vi "AlliGator Fit Method Benchmark.vi"() -> ()   [LabVIEW 2021, in "AlliGator Fit Method Benchmark.lvlib"]
doc: "Fit Method Benchmark GUI."
uses:
  AlliGator Fit Method Benchmark.lvlib
  AlliGator Fit Simulation Parameters.ctl
  AlliGator Decay Simulation Parameters.ctl
  Arrays/Array Statistics.ctl
  Fits/IRF(X)PSED/Decay Fit Options v4.ctl
  Fits/Decay Convolution/Decay Model.ctl
  Fits/Residual Type.ctl
  Fits/IRF(X)PSED/Fit Weights Type v2.ctl
  Fits/Non-linear Fitting Method v2.ctl
  Fits/Fit Calculation Method.ctl
  Fits/Non-linear Fitting Algorithm.ctl
  Decay Analysis/Decay Fit/AlliGator Decay Fit Parameter Constraints 2.ctl
  Fits/IRF(X)PSED/Decay Fit Parameters In List.ctl
  Fits/IRF(X)PSED/MLE Baseline Offset Type.ctl
  AlliGator Simulation Parameters.ctl
  AlliGator Simulation Parameters x Factors.ctl
  AlliGator FMB Histogram Options.ctl
  Graphs/XY Graph/XY Graph Refnum.ctl
  AlliGator FMB Q Element.ctl
  AlliGator FMB Q Event List.ctl
  AlliGator Simulation & Fit Options & Parameters.ctl
  Decay Fit Parameter Map/AlliGator Decay Fit Options & Parameters v4.ctl
  Graphs/XY Graph/XY Graph Event.ctl
  <vilib>/Utility/miscctls.llb/LVPoint32TypeDef.ctl
  Rich Text Box/Text Format List.ctl
  AlliGator FMB Output.ctl
  1fb6a2ff-6d04-4407-a86c-ead387429d5f.vi
  8e253123-243f-4246-a918-c0cefae78a39.vi
  91ed939d-9414-4ac9-84f6-330e4a8e3c9b.vi
  AlliGator FMB Global.vi
  Variant/Variant to Data/Variant to DBL.vi
  Graphs/XY Graph/XY Graph Add Single Plot with Name.vi
  Variant/Variant to Data/Variant to I32.vi
  GUI/GUI.lvlib
  Notebook/Notebook.lvlib
  Error/Error.lvlib
  Graphs/XY Graph/XY Graph Add-Ons.lvlib
  Utilities/Utilities.lvlib
  Fits/Fits.lvlib
  Decay Analysis/Decay Fit/AlliGator Decay Fit.lvlib
  <vilib>/vision/NI_Vision_Development_Module.lvlib
  Variant/Variant to Data/Variant to Data.lvlib
  Strings/Strings.lvlib
  Arrays/Arrays.lvlib
  Decay Fit Parameter Map/AlliGator Decay Fit Parameter Map.lvlib
panel:
  in  "Tab Control":T1(tab)
  in  "Histogram Options":T2={"Histogram Bin Size (Lifetime)"=1.0000000000000002e-10, "Histogram Bin Size (a1)"=0.1, "Histogram Upper Percentile"=100.0, "Histogram Lower Percentile"=0.0, "Histogram Fit"=FALSE}
  out "Histograms ToolTip":string
  in  "Export Results":bool
  out "Histograms":cluster{"Axis":dbl[], "Histogram":dbl[]}[](graph)
  in  "Run Simulation":bool
  in  "Fit Simulation Parameters":T3={"# Counts"=100, "# Simulations (N)"=100, "Decay Bin Size"=1.0000000000000002e-10, "# Bins"=200}
  in  "Decay Simulation Parameters":T4={"tau 1"=1e-09, "tau 2"=0.0, "a1"=1.0, "Baseline"=0.0}
  out "tau 1":T5 {"Min" format="%#_4g"; "Max" format="%#_4g"; "Mean" format="%#_4g"; "Standard Deviation" format="%#_4g"}
  out "tau 2":T5 {"Min" format="%#_4g"; "Max" format="%#_4g"; "Mean" format="%#_4g"; "Standard Deviation" format="%#_4g"}
  out "a1":T5 {"Min" format="%#_4g"; "Max" format="%#_4g"; "Mean" format="%#_4g"; "Standard Deviation" format="%#_4g"}
  out "Simulation Summary":string caption="Output (see Notebook)"
  out "Decay Graph ToolTip":string
  out "# Photons":dbl[](array[numeric])
  in  "Select Decay, Fit & Residuals Index":i32=1 min=1
  out "Decay Graph":cluster{"Axis":dbl[], "Histogram":dbl[]}[](graph)
  in  "Plot Decays, Fits & Residuals":bool
  out "Experimental IRF Loaded":bool
  in  "Use Experimental IRF":bool
  in  "# Logical Processors Used":i32=4 caption="Used" min=1 max=16
  out "# Logical Processors":i32
  in  "MLE Baseline Offset Type":T6
  in  "MLE Baseline Offset":dbl
  in  "Fit Parameter Constraints":T7[](array[typedef]) {"Max Value" format="%#.3g"; "Min Value" format="%#.3g"}
  in  "Decay Fit Options":T9={"Show Fit Residuals"=TRUE, "Fit Model"=enum."1-Exponential", "Residual Type"=enum."Normalized", "Max Decay Percentile"=100.0, "Min Decay Percentile"=0.0, "Show Full Decay"=TRUE, "Weights"=enum."Unweighted", "Fitting Method"=enum."Least Square", "Compute Parameter Uncertainties"=TRUE, "Periodic Boundaries"=TRUE, "Model Calculation"=enum."Convolution", "Period"=1.2500000000000001e-08, "Termination Criteria"={"Max Iterations"=1000, "Max Function Calls"=10000, "Max Time"=100.0, "Function Tolerance"=1e-09, "Parameter Tolerance"=1e-09, "Gradient Tolerance"=1e-09, "Min Lambda"=1e-09, "Max Lambda"=1000000000.0, "Initial Tick Count"=0}, "Offset Resolution"=5.000000000000001e-11, "Use Local IRF"=FALSE, "Fitting Algorithm"=enum."Levenberg-Marquardt", "Show Confidence Interval "=FALSE, "Confidence Level"=95.0} {"Confidence Level" min=0.0 max=100.0; "Offset Resolution" min=0.0; "Period" min=0.0; "Min Decay Percentile" min=0.0 max=1.0; "Max Decay Percentile" min=0.0 max=100.0}
  in  "# Steps":i32
  in  "Run Script":bool
  in  "Simulation Parameters Multiplication Factor (s)":T16={"Decay Simulation Parameters"={"tau 1"=1.0, "tau 2"=1.0, "a1"=1.0, "Baseline"=1.0}, "Fit Simulation Parameters"={"# Counts"=1.0, "# Simulations (N)"=1.0, "Decay Bin Size"=1.0, "# Bins"=1.0}} {"Fit Simulation Parameters"."# Bins" format="%#_5f"; "Fit Simulation Parameters"."# Simulations (N)" format="%#_5f"; "Fit Simulation Parameters"."# Counts" format="%#_5f"}
  in  "Simulation Parameters Increment(s)":T17
  in  "Parameter Set Choice":T18(radio)
  in  "Simulation Parameters":T17[](array[typedef])
  in  "Animated Busy Icon":bool=TRUE
  in  "Abort":bool
  out "Progress Bar":dbl(slide) scale=0.0..100.0
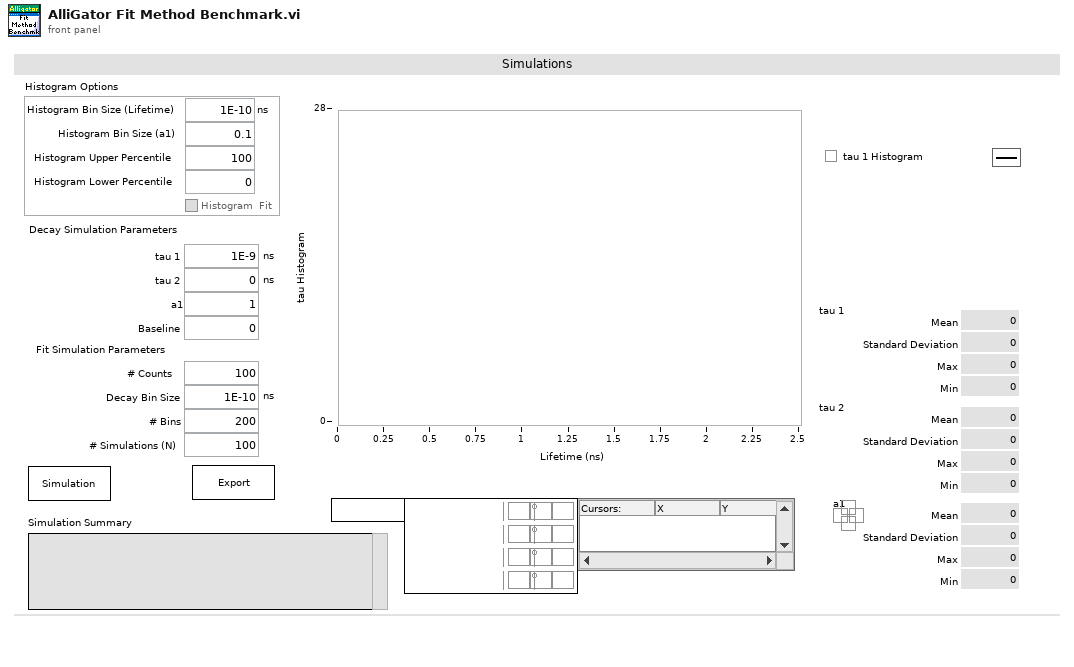
[diagram p1: front panel]
types:
  T1 = enum32{"Simulations", "Decay, Fit & Residuals Plots", "Settings", "Scripts"}
  T2 = typedef "AlliGator Fit Method Benchmark.lvlib/AlliGator FMB Histogram Options.ctl" = cluster{"Histogram Bin Size (Lifetime)":dbl[unit], "Histogram Bin Size (a1)":dbl, "Histogram Upper Percentile":dbl, "Histogram Lower Percentile":dbl, "Histogram Fit":bool}
  T3 = typedef "AlliGator Fit Method Benchmark.lvlib/AlliGator Fit Simulation Parameters.ctl" = cluster{"# Counts":i32, "# Simulations (N)":i32, "Decay Bin Size":dbl[unit], "# Bins":i32}
  T4 = typedef "AlliGator Fit Method Benchmark.lvlib/AlliGator Decay Simulation Parameters.ctl" = cluster{"tau 1":dbl[unit], "tau 2":dbl[unit], "a1":dbl, "Baseline":dbl}
  T5 = typedef "Arrays.lvlib/Array Statistics.ctl" = cluster{"Mean":dbl, "Standard Deviation":dbl, "Max":dbl, "Min":dbl}
  T6 = typedef "Fits.lvlib/MLE Baseline Offset Type.ctl" = enum32{"Absolute", "Percentage"}
  T7 = typedef "AlliGator Decay Fit.lvlib/AlliGator Decay Fit Parameter Constraints 2.ctl" = cluster{"Fit Parameter":T8, "Min Value":dbl, "Max Value":dbl, "Global":bool, "Used":bool}
  T8 = typedef "Fits.lvlib/Decay Fit Parameters In List.ctl" = enum16{"Offset", "Baseline", "A_1", "tau_1", "A_2", "tau_2"}
  T9 = typedef "Fits.lvlib/Decay Fit Options v4.ctl" = cluster{"Show Fit Residuals":bool, "Fit Model":T10, "Residual Type":T11, "Max Decay Percentile":dbl, "Min Decay Percentile":dbl, "Show Full Decay":bool, "Weights":T12, "Fitting Method":T13, "Compute Parameter Uncertainties":bool, "Periodic Boundaries":bool, "Model Calculation":T14, "Period":dbl[unit], "Termination Criteria":cluster{"Max Iterations":i32, "Max Function Calls":i32, "Max Time":dbl[unit], "Function Tolerance":dbl, "Parameter Tolerance":dbl, "Gradient Tolerance":dbl, "Min Lambda":dbl, "Max Lambda":dbl, "Initial Tick Count":u32}, "Offset Resolution":dbl[unit], "Use Local IRF":bool, "Fitting Algorithm":T15, "Show Confidence Interval ":bool, "Confidence Level":dbl}
  T10 = typedef "Fits.lvlib/Decay Model.ctl" = enum16{"1-Exponential", "2-Exponentials"}
  T11 = typedef "Fits.lvlib/Residual Type.ctl" = enum16{"Standard", "Normalized", "Reduced"}
  T12 = typedef "Fits.lvlib/Fit Weights Type v2.ctl" = enum16{"Unweighted", "1/Variance (Neyman)", "1/Variance (Pearson)", "Best of All"}
  T13 = typedef "Fits.lvlib/Non-linear Fitting Method v2.ctl" = enum16{"Least Square", "Least Absolute Residual", "Bisquare", "MLE", "-", "Best of All"}
  T14 = typedef "Fits.lvlib/Fit Calculation Method.ctl" = enum16{"Simulation", "Convolution", "Integration"}
  T15 = typedef "Fits.lvlib/Non-linear Fitting Algorithm.ctl" = enum16{"Levenberg-Marquardt", "Trust-Region Dogleg"}
  T16 = typedef "AlliGator Fit Method Benchmark.lvlib/AlliGator Simulation Parameters x Factors.ctl" = cluster{"Decay Simulation Parameters":cluster{"tau 1":dbl, "tau 2":dbl, "a1":dbl, "Baseline":dbl}, "Fit Simulation Parameters":cluster{"# Counts":dbl, "# Simulations (N)":dbl, "Decay Bin Size":dbl, "# Bins":dbl}}
  T17 = typedef "AlliGator Fit Method Benchmark.lvlib/AlliGator Simulation Parameters.ctl" = cluster{"Decay Simulation Parameters":T4, "Fit Simulation Parameters":T3, "Use Experimental IRF":bool}
  T18 = enum32{"User-provided Array", "Parameter Increment", "Parameter x Factor"}
  T19 = typedef "AlliGator Fit Method Benchmark.lvlib/AlliGator Simulation & Fit Options & Parameters.ctl" = cluster{"Simulation Parameters":T17, "Decay Fit Options & Parameters":T20}
  T20 = typedef "AlliGator Decay Fit Parameter Map.lvlib/AlliGator Decay Fit Options & Parameters v4.ctl" = cluster{"SYNC Period":dbl[unit], "Fit Options":T9, "Fit Parameter Constraints":T7[], "MLE Baseline Offset":dbl, "MLE Baseline Offset Type":T6}
  T21 = typedef "AlliGator Fit Method Benchmark.lvlib/AlliGator FMB Q Event List.ctl" = enum16{"Idle", "Initialization", "Update Script Simulation Parameters", "Single Simulation Prelude", "Run Simulation", "Update Histograms", "Update Script Simulation Output", "Graph Event", "Show Selected Decay", "Export Results", "Update # Processors Used", "Check Baseline", "Run Script", "End Script", "Init", "Abort", "Quit"}
  T22 = typedef "AlliGator Fit Method Benchmark.lvlib/AlliGator FMB Q Element.ctl" = cluster{"FMB Q Event":T21, "Data":variant}
  T23 = cluster{"Decay Graph":refnum<event-registration>, "Histograms":refnum<event-registration>}
  T24 = typedef "XY Graph Add-Ons.lvlib/XY Graph Refnum.ctl" = refnum<vi>
  T25 = typedef "XY Graph Add-Ons.lvlib/XY Graph Event.ctl" = cluster{"Item Tag":string, "XY Graph Refnum":refnum<vi>, "Coords":T26, "Item Path":string}
  T26 = typedef "LVPoint32TypeDef.ctl" = cluster{"Horizontal":i32, "Vertical":i32}
  T27 = typedef "Notebook.lvlib/Text Format List.ctl" = enum16{"Message", "Result", "Error", "Setting", "Verbose", "Warning"}
  T28 = typedef "AlliGator Fit Method Benchmark.lvlib/AlliGator FMB Output.ctl" = cluster{"Simulation & Fit Options & Parameters":T19, "Array Statistic (tau 1)":T5, "Array Statistics (a1)":T5, "Array Statistics (tau 2)":T5}
  T29 = cluster{"Decay Fit Options":T9, "Fit Parameter Constraints":T7[], "Use Experimental IRF":bool, "MLE Baseline Offset Type":T6, "MLE Baseline Offset":dbl}
  T30 = typedef "XY Graph Add-Ons.lvlib/XY Graph Plot Data.ctl" = cluster{"X Array":dbl[], "Y Array":dbl[]}
  T31 = typedef "Fits.lvlib/IRF(X)PSED Fit Results.ctl" = cluster{"Best Fit Parameters (All)":dbl[], "Delta Best Fit Parameters (All)":dbl[], "R^2":dbl, "Reduced Chi^2":dbl}
  T32 = typedef "Rich Text Box.lvlib/Text Formatting.ctl" = cluster{"Font":string, "Text Color":T33, "Background Color":T33, "Style":T34, "Font Size":dbl, "Alignment":T35}
  T33 = typedef "Rich Text Box.lvlib/Text Colors.ctl" = enum16{"Unchanged", "Black", "Blue", "Cyan", "Maroon", "Gray", "Violet", "Green", "Light Green", "Orange", "Yellow", "Magenta", "Red", "White"}
  T34 = typedef "Rich Text Box.lvlib/Text Style.ctl" = enum16{"Regular", "Bold", "Italic", "Underline", "Strikeout"}
  T35 = typedef "Rich Text Box.lvlib/Text Alignment.ctl" = enum16{"Left", "Right", "Center"}
  T36 = typedef "AlliGator Progress Bar Q Element.ctl" = cluster{"Action":string, "Value":dbl}
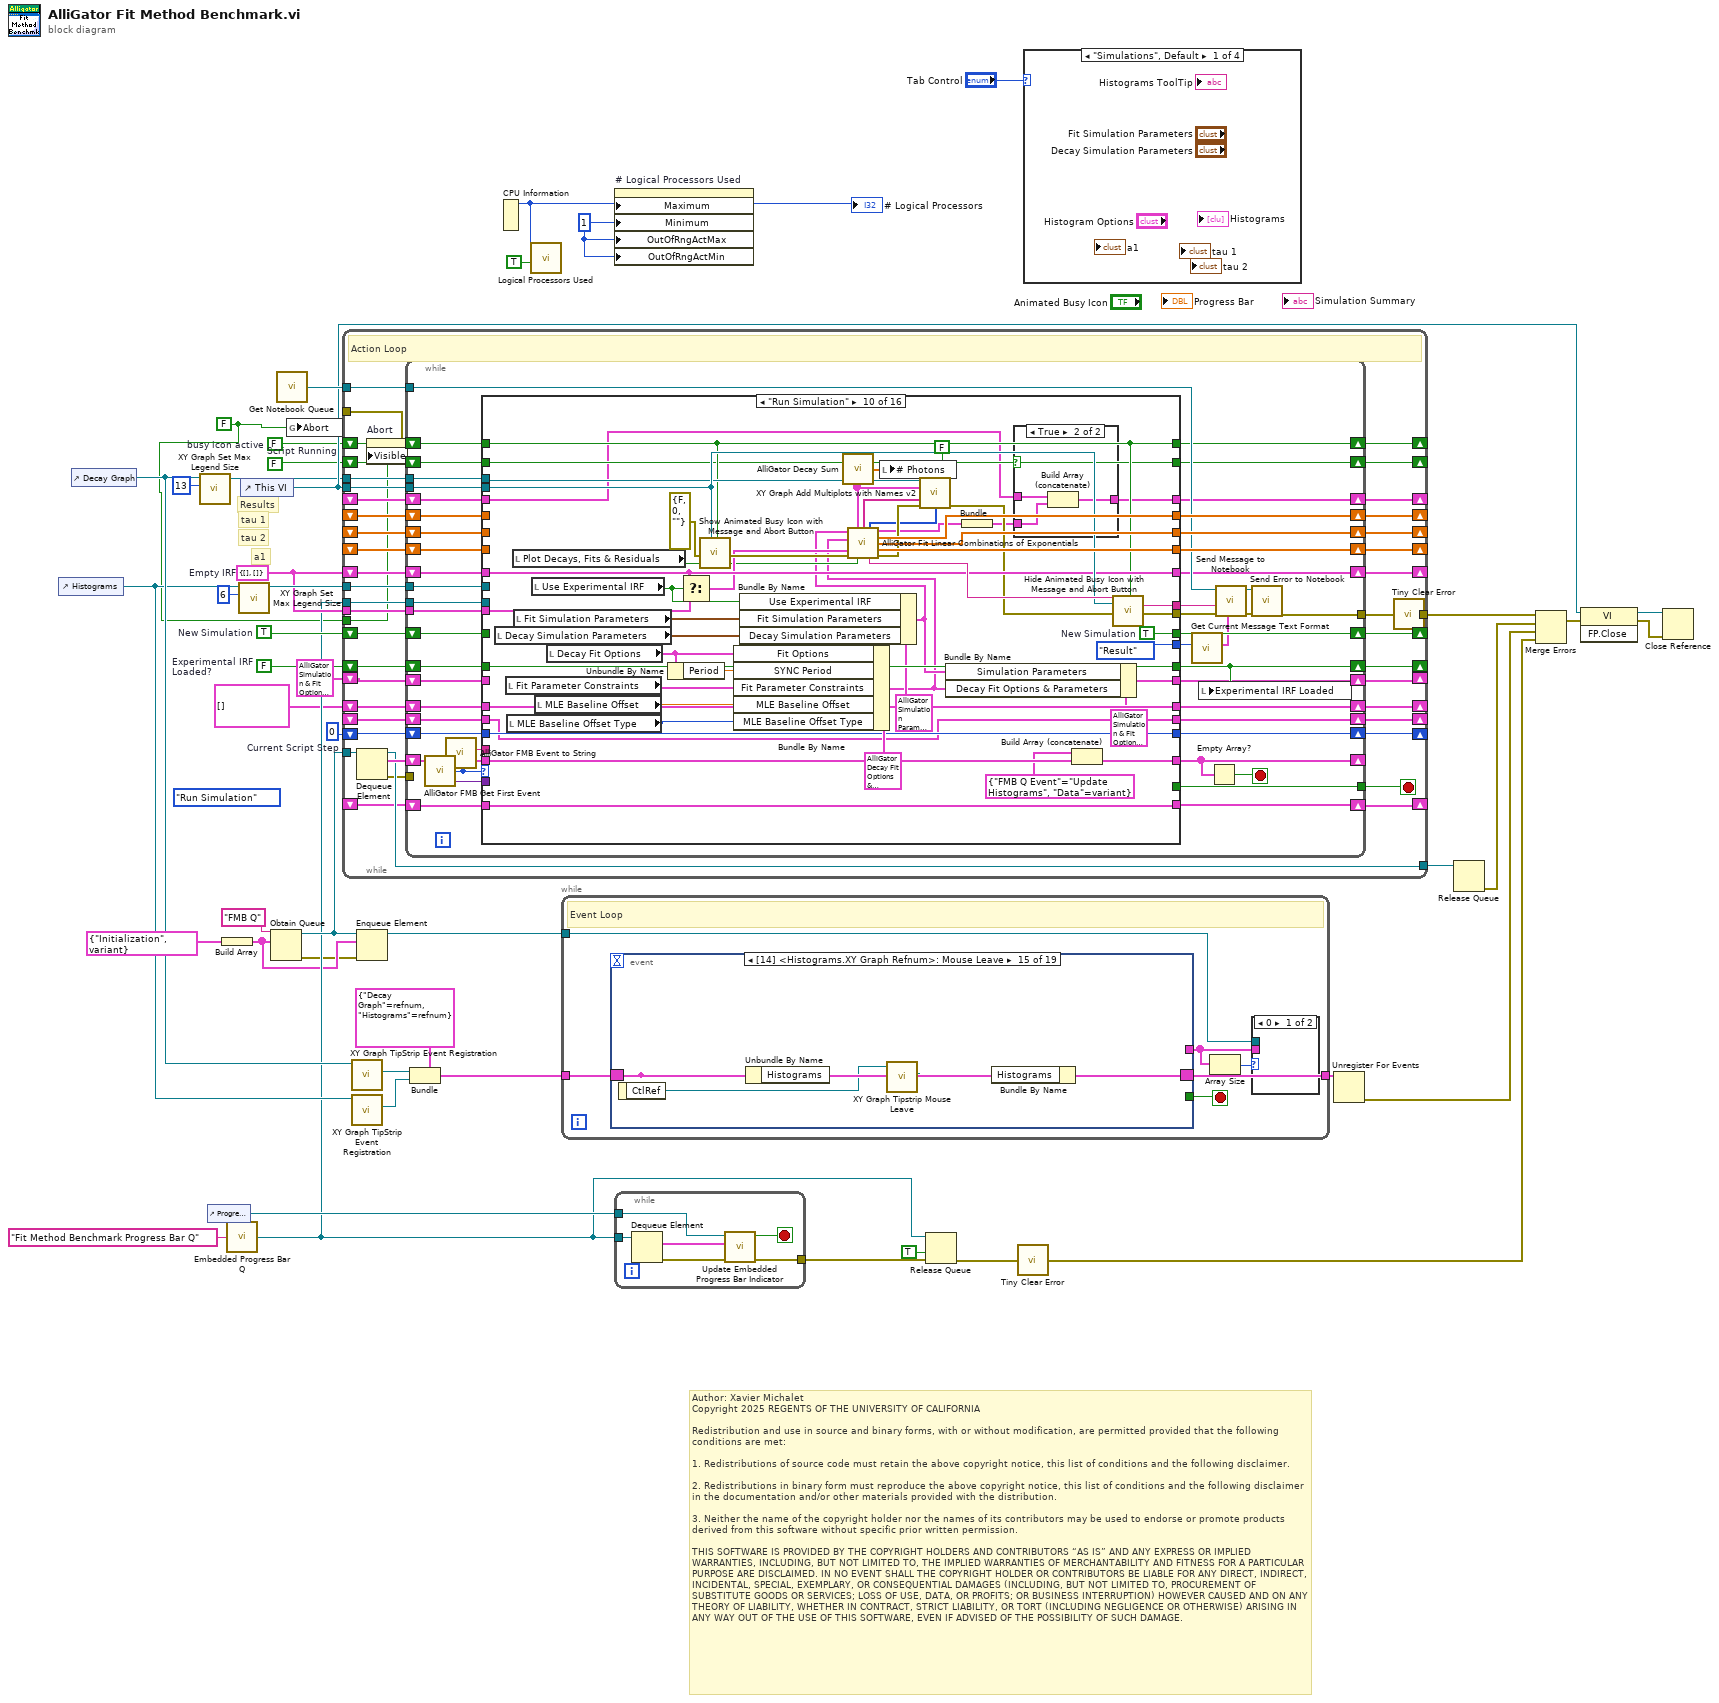
[diagram p0: block diagram]
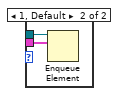
[diagram p2: hidden frame]
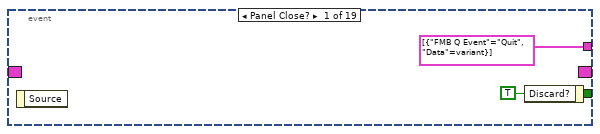
[diagram p3: hidden frame]
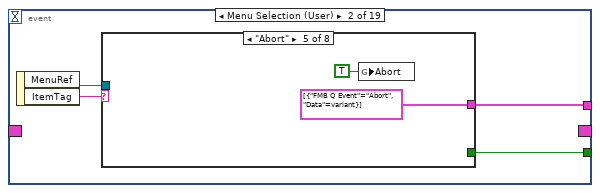
[diagram p4: hidden frame]
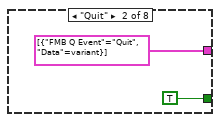
[diagram p6: hidden frame]
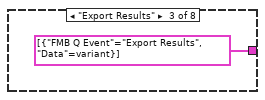
[diagram p7: hidden frame]
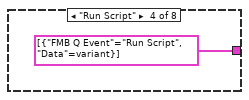
[diagram p8: hidden frame]
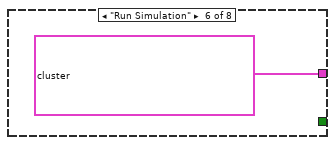
[diagram p9: hidden frame]
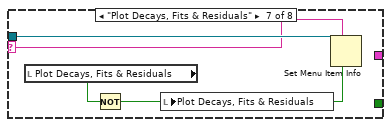
[diagram p10: hidden frame]
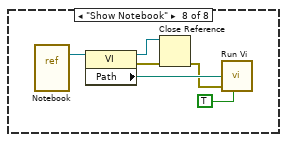
[diagram p11: hidden frame]
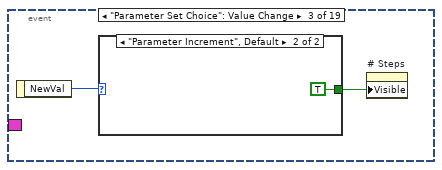
[diagram p12: hidden frame]
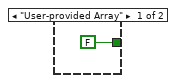
[diagram p13: hidden frame]
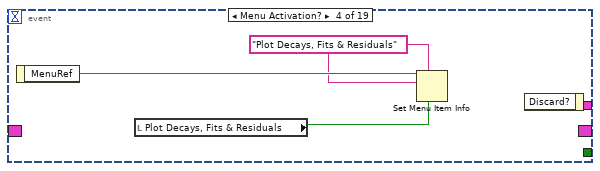
[diagram p14: hidden frame]
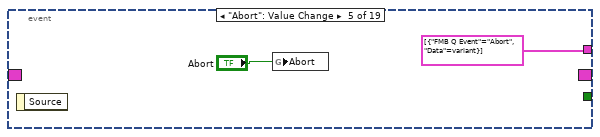
[diagram p15: hidden frame]
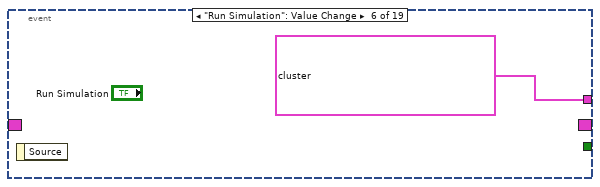
[diagram p16: hidden frame]
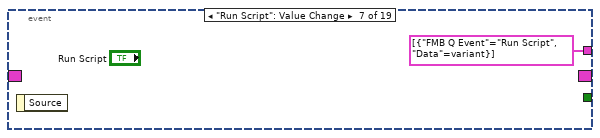
[diagram p17: hidden frame]
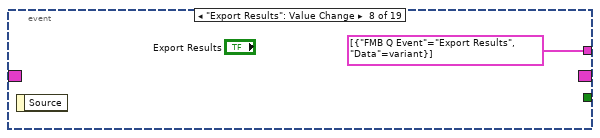
[diagram p18: hidden frame]
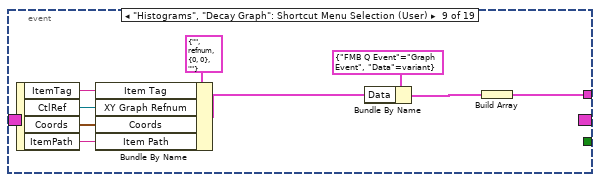
[diagram p19: hidden frame]
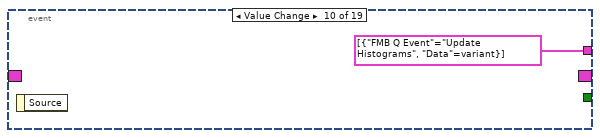
[diagram p20: hidden frame]
diagram:
  w6 = 0  # Current Script Step
  w7 = FALSE  # Script Running
  (unwired) AlliGator_FMB_Q_Event_List."Run Simulation" ("Named Q Event")
  w19 = FALSE  # busy icon active
  w26 = FALSE  # Experimental IRF Loaded?
  w27 = cluster{"t Array":dbl[], "IRF Array":dbl[]} {"t Array"=[], "IRF Array"=[]}  # Empty IRF
  w28 = u8 1 ("Data Entry Limits:Minimum")
  w31 = TRUE  # New Simulation
  w1 = FALSE ("Visible")
  # "Author: Xavier Michalet\nCopyright 2025 REGENTS OF THE UNIVERSITY OF CALIFORNIA\n\nRedistribution and use in source and binary forms, with or without modification, are permitted provided that the following conditions are met:\n\n1. Redistributions of source code must retain the above copyright notice, this list of conditions and the following disclaimer.\n\n2. Redistributions in binary form must reproduce the above copyright notice, this list of conditions and the following disclaimer in the documentation and/or other materials provided with the distribution.\n\n3. Neither the name of the copyright holder nor the names of its contributors may be used to endorse or promote products derived from this software without specific prior written permission.\n\nTHIS SOFTWARE IS PROVIDED BY THE COPYRIGHT HOLDERS AND CONTRIBUTORS “AS IS” AND ANY EXPRESS OR IMPLIED WARRANTIES, INCLUDING, BUT NOT LIMITED TO, THE IMPLIED WARRANTIES OF MERCHANTABILITY AND FITNESS FOR A PARTICULAR PURPOSE ARE DISCLAIMED. IN NO EVENT SHALL THE COPYRIGHT HOLDER OR CONTRIBUTORS BE LIABLE FOR ANY DIRECT, INDIRECT, INCIDENTAL, SPECIAL, EXEMPLARY, OR CONSEQUENTIAL DAMAGES (INCLUDING, BUT NOT LIMITED TO, PROCUREMENT OF SUBSTITUTE GOODS OR SERVICES; LOSS OF USE, DATA, OR PROFITS; OR BUSINESS INTERRUPTION) HOWEVER CAUSED AND ON ANY THEORY OF LIABILITY, WHETHER IN CONTRACT, STRICT LIABILITY, OR TORT (INCLUDING NEGLIGENCE OR OTHERWISE) ARISING IN ANY WAY OUT OF THE USE OF THIS SOFTWARE, EVEN IF ADVISED OF THE POSSIBILITY OF SUCH DAMAGE."
  # "Results"
  # "a1"
  # "tau 2"
  # "tau 1"
  n1 = control-ref of="Histograms"() -> (w23:refnum<vi>)
  n2 = control-ref of="Decay Graph"() -> (w24:refnum<vi>)
  n3 = call "XY Graph Set Max Legend Size.vi"("Max Legend Size"=13, "XY Graph Refnum"=w24) -> ("XY Graph Refnum (dup)"=w33:T24)  [unwired: 8 in, 1 out]
  n4 = control-ref of="Progress Bar"() -> (w45:refnum<vi>)
  n5 = Build Array(T22 {"FMB Q Event"=enum."Initialization", "Data"=variant} ("FMB Q Element")) -> (w4:T22[])
  n6 = call "Embedded Progress Bar Q.vi"("Progress Bar Queue Name"="Fit Method Benchmark Progress Bar Q") -> ("Progress Bar Queue"=w9:refnum<queue>)  [unwired: 6 in]
  n7 = call "XY Graph Set Max Legend Size.vi"("Max Legend Size"=6, "XY Graph Refnum"=w23) -> ("XY Graph Refnum (dup)"=w34:T24)  [unwired: 8 in, 1 out]
  n8 = control-ref of="This VI"() -> (w36:refnum<vi>)
  n9 = Obtain Queue(name (unnamed)="FMB Q", element data type=w4) -> (queue out=w15:refnum<queue>, error out=w3:errorcluster)  [unwired: 3 in, 1 out]
  n10 = call "Get Notebook Queue.vi"() -> ("Notebook Queue"=w42:refnum<queue>)  [unwired: 9 in]
  n11 = global write "AlliGator FMB Global.vi" "Abort"(w1) -> ()
  n12 = while {
    shift-right: [w88] -> _
    shift-left: _ -> [w85]
    shift-right: [w87] -> _
    shift-left: _ -> [w84]
    shift-right: [w86] -> _
    shift-left: _ -> [w83]
    tunnel: w9 -> [w82]
    tunnel: w42 -> [w81]
    tunnel: [w79] -> w41
    tunnel: [w47] -> _
    tunnel: w36 -> [w78]
    tunnel: w34 -> [w77]
    shift-right: [w76] -> _
    shift-left: _ -> [w75]
    tunnel: w33 -> [w74]
    shift-right: [w72] -> _
    shift-left: w31 -> [w73]
    shift-right: [w70] -> _
    shift-left: w27 -> [w71]
    tunnel: w27 -> [w69]
    shift-right: [w65] -> _
    shift-left: w26 -> [w68]
    shift-right: [w66] -> _
    shift-left: w19 -> [w67]
    tunnel: w15 -> [w64]
    tunnel: [w62] -> w12
    shift-right: [w61] -> _
    shift-left: T17[] [] ("Simulation Parameters Array") -> [w60]
    shift-right: [w57] -> _
    shift-left: w7 -> [w58]
    shift-right: [w55] -> _
    shift-left: w6 -> [w56]
    shift-right: [w50] -> _
    shift-left: _ -> [w49]
    shift-right: [w54] -> _
    shift-left: T19 {"Simulation Parameters"={"Decay Simulation Parameters"={"tau 1"=0.0, "tau 2"=0.0, "a1"=0.0, "Baseline"=0.0}, "Fit Simulation Parameters"={"# Counts"=0, "# Simulations (N)"=0, "Decay Bin Size"=0.0, "# Bins"=0}, "Use Experimental IRF"=FALSE}, "Decay Fit Options & Parameters"={"SYNC Period"=0.0, "Fit Options"={"Show Fit Residuals"=FALSE, "Fit Model"=enum."1-Exponential", "Residual Type"=enum."Standard", "Max Decay Percentile"=0.0, "Min Decay Percentile"=0.0, "Show Full Decay"=FALSE, "Weights"=enum."Unweighted", "Fitting Method"=enum."Least Square", "Compute Parameter Uncertainties"=FALSE, "Periodic Boundaries"=FALSE, "Model Calculation"=enum."Simulation", "Period"=0.0, "Termination Criteria"={"Max Iterations"=0, "Max Function Calls"=0, "Max Time"=0.0, "Function Tolerance"=0.0, "Parameter Tolerance"=0.0, "Gradient Tolerance"=0.0, "Min Lambda"=0.0, "Max Lambda"=0.0, "Initial Tick Count"=0}, "Offset Resolution"=0.0, "Use Local IRF"=FALSE, "Fitting Algorithm"=enum."Levenberg-Marquardt", "Show Confidence Interval "=FALSE, "Confidence Level"=0.0}, "Fit Parameter Constraints"=[], "MLE Baseline Offset"=0.0, "MLE Baseline Offset Type"=enum."Absolute"}} ("output cluster") -> [w53]
    shift-right: [w52] -> _
    shift-left: _ -> [w51]
    tunnel: w1 -> [w48]
    stop <- w89 stop-if-true
    # "Action Loop"
    n13 = Dequeue Element(queue=w64) -> (queue out=w62:refnum<queue>, element=w63:T22[], error out=w59:errorcluster)  [unwired: 2 in, 1 out]
    n14 = property on="Abort" class="Bool"("Visible"=w48) -> (error out=w47:errorcluster)  [unwired: 2 in, 1 out]
    n15 = while {
      tunnel: [w138] -> w89
      tunnel: w82 -> [w131]
      tunnel: w81 -> [w130]
      tunnel: [w126] -> w80
      tunnel: w78 -> [w124]
      tunnel: w77 -> [w123]
      tunnel: w74 -> [w120]
      tunnel: w69 -> [w115]
      shift-right: [w118] -> w72
      shift-left: w73 -> [w119]
      shift-right: [w109] -> w65
      shift-left: w68 -> [w114]
      shift-right: [w110] -> w66
      shift-left: w67 -> [w111]
      shift-right: [w104] -> _
      shift-left: w63 -> [w108]
      shift-right: [w122] -> w76
      shift-left: w75 -> [w121]
      shift-right: [w137] -> w88
      shift-left: w85 -> [w134]
      shift-right: [w136] -> w87
      shift-left: w84 -> [w133]
      shift-right: [w135] -> w86
      shift-left: w83 -> [w132]
      shift-right: [w116] -> w70
      shift-left: w71 -> [w117]
      shift-right: [w103] -> w61
      shift-left: w60 -> [w102]
      tunnel: w59 -> [_]
      shift-right: [w99] -> w57
      shift-left: w58 -> [w98]
      shift-right: [w96] -> w55
      shift-left: w56 -> [w97]
      shift-right: [w91] -> w50
      shift-left: w49 -> [w90]
      shift-right: [w95] -> w54
      shift-left: w53 -> [w94]
      shift-right: [w93] -> w52
      shift-left: w51 -> [w92]
      stop <- w106 stop-if-true
      n16 = call "AlliGator FMB Get First Event.vi"("Named Q Elements"=w108) -> ("Data"=w107:variant, "Named Q Event"=w101:T21, "Named Q Elements"=w105:T22[])  [unwired: 2 in]
      n17 = call "AlliGator FMB Event to String.vi"("FMB Q Event"=w101) -> ("String"=w100:string)  [unwired: 8 in]
      n18 = case shown="\"Run Simulation\"" w101 {
        tunnel: [_ _ _ _ _ _ _ TRUE ("Discard?") _ _ _ _ _ _ _ _] -> w138
        tunnel: [w158 w178 w201 w224 w249 w282 w306 w319 w348 w411 w440 w459 w478 w507 w559 w576] -> w137
        tunnel: [w157 w177 w200 w223 w248 w281 w305 w319 w347 w410 w439 w458 w477 w506 w558 w575] -> w136
        tunnel: [w156 w176 w199 w222 w247 w280 w304 w319 w346 w409 w438 w457 w476 w505 w557 w574] -> w135
        tunnel: w134 -> [w158 w178 w201 w224 w249 w282 w306 _ w348 _ w440 w459 w478 w507 w559 w576]
        tunnel: w133 -> [w157 w177 w200 w223 w248 w281 w305 _ w347 _ w439 w458 w477 w506 w558 w575]
        tunnel: w132 -> [w156 w176 w199 w222 w247 w280 w304 _ w346 _ w438 w457 w476 w505 w557 w574]
        tunnel: w131 -> [_ _ _ _ _ _ _ w318 _ _ _ _ _ _ _ _]
        tunnel: [w150 _ w189 w212 w246 _ _ _ w331 w408 _ _ _ w504 _ _] -> w129
        tunnel: [w149 _ w185 w221 w245 _ _ _ w330 w407 _ _ _ w503 _ _] -> w125
        tunnel: w124 -> [w145 _ w188 _ _ _ _ _ w328 w406 _ _ _ _ _ _]
        tunnel: w123 -> [_ _ _ _ _ _ _ _ _ _ _ _ _ w502 _ _]
        tunnel: [w155 w175 w198 w220 w244 w284 w303 _ _ w375 w437 w456 w475 w501 w556 w573] -> w122
        tunnel: w121 -> [w155 w175 w198 w220 w244 w284 w303 _ _ w374 w437 w456 w475 w501 w556 w573]
        tunnel: w120 -> [_ _ _ _ _ _ _ _ _ w405 w436 _ _ _ _ _]
        tunnel: w119 -> [w154 w174 w197 w219 w243 w278 w302 w317 w345 _ w435 w455 w474 w500 w555 w572]
        tunnel: [w154 w174 w197 w219 w243 w278 w302 w317 w345 w404 w435 w455 w474 FALSE ("New Simulation") w555 w572] -> w118
        tunnel: w117 -> [w153 w173 w196 w218 w242 w279 w301 w316 w344 w403 w434 w454 w473 w498 w554 w571]
        tunnel: [w153 w173 w196 w218 w241 w279 w301 w316 w344 w403 w434 w454 w473 w498 w554 w571] -> w116
        tunnel: w115 -> [_ _ _ _ _ _ _ _ _ w402 _ _ _ _ _ _]
        tunnel: w114 -> [w152 w171 w195 w216 w240 w277 w299 w314 w343 w400 w432 w452 w471 w495 w552 w569]
        tunnel: [_ _ _ _ w232 _ _ _ _ Text_Format_List."Result" ("Text Format") _ _ _ Text_Format_List."Result" ("Text Format") _ _] -> w112
        tunnel: w111 -> [_ w172 _ w217 w239 w283 w300 w315 _ w380 w433 w453 w472 w496 w553 w570]
        tunnel: [w143 w172 w179 w217 w239 w283 w300 w315 w326 w380 w433 w453 w472 w496 w553 w570] -> w110
        tunnel: [w152 w171 w195 w216 w238 w277 w299 w314 w343 w400 w432 w452 w471 w495 w552 w569] -> w109
        tunnel: w107 -> [_ w167 _ _ w237 _ _ _ _ _ w423 _ w468 _ _ _]
        tunnel: w105 -> [_ w165 w194 w215 w231 w285 w298 _ w335 w384 w424 w451 w466 w487 w551 w568]
        tunnel: [T22[] [] ("Named Q Elements") w165 w194 w215 w231 w285 w298 T22[] [] ("Named Q Elements") w334 w383 w424 w451 w466 w487 w551 w568] -> w104
        tunnel: [w151 w164 w193 w206 w230 w276 w297 w313 w333 w382 w422 w447 w465 w486 w546 w567] -> w103
        tunnel: w102 -> [w151 w164 w193 w206 w230 w276 w297 w313 _ w382 w422 _ w465 w486 w546 w567]
        tunnel: w100 -> [_ _ _ _ _ _ _ _ w327 _ _ _ _ _ _ _]
        tunnel: [w143 w163 w179 w214 w229 w275 w296 w311 w326 w378 w421 w450 w464 w485 w547 w566] -> w99
        tunnel: w98 -> [_ w163 _ w214 w229 w275 w296 w311 _ w378 w421 w450 w464 w485 w547 w566]
        tunnel: w97 -> [w142 w162 w186 w213 w228 w274 w295 w310 _ w373 w420 _ w463 w484 w542 w561]
        tunnel: [w142 w162 w186 w213 w228 w274 w295 w310 0 w373 w420 0 ("Current Script Step") w463 w484 w542 w560] -> w96
        tunnel: [w141 w161 w183 w204 w227 w273 w288 w309 w323 w365 w419 w443 w462 w483 w545 w565] -> w95
        tunnel: w94 -> [w141 w161 w183 w204 w227 w273 w288 w309 w323 _ w419 w443 w462 w483 w545 w565]
        tunnel: [w140 w160 w182 w203 w226 w272 w287 w308 w322 w364 w418 w442 w461 w482 w544 w562] -> w93
        tunnel: w92 -> [w140 w160 w182 w203 w226 w272 w287 w308 w322 w364 w418 w442 w461 w481 w544 w562]
        tunnel: [w139 w159 w181 w202 w225 w271 w286 w307 w321 w363 w417 w441 w460 w480 w543 w563] -> w91
        tunnel: w90 -> [w139 w159 w181 w202 w225 w271 w286 w307 _ w363 w417 w441 w460 w480 w543 w564]
        frame "Abort" {
          w143 = FALSE ("Visible")
          n19 = call "Hide Animated Busy Icon with Message and Abort Button.vi"("Target VI reference"=w145) -> ()  [unwired: 18 in, 1 out]
          n20 = call "Current Date & Time String.vi"() -> ("time string"=w147:string, "date string"=w148:string)  [unwired: 9 in, 1 out]
          n21 = Format Into String(format string="Script aborted on %s at %s.", w148, w147) -> (resulting string=w150:string, error out=w149:errorcluster)  [unwired: 2 in]
        }
        frame "Check Baseline" {
          n22 = call-poly "Variant to Data.vi"("Variant"=w167) -> ("Value"=w166:dbl)  [unwired: 8 in]
          n23 = property on="# Bins" class="DigNum (strict)"() -> ("Value"=w170:i32)  [unwired: 2 in, 2 out]
          n24 = property on="# Counts" class="DigNum (strict)"() -> ("Value"=w169:i32)  [unwired: 2 in, 2 out]
          n25 = call "AlliGator Baseline Simulation Check.vi"("# Counts"=w169, "# Bins"=w170, "New Baseline in"=w166) -> ("New Baseline out"=w168:dbl)  [unwired: 8 in]
          n26 = property on="Baseline" class="DigNum (strict)"("Value"=w168) -> ()  [unwired: 2 in, 2 out]
        }
        frame "End Script" {
          w179 = FALSE ("Visible")
          n27 = call "Hide Animated Busy Icon with Message and Abort Button.vi"("Target VI reference"=w188) -> ("Error Out"=w187:errorcluster)  [unwired: 18 in]
          n28 = call "Current Date & Time String.vi"("Error In"=w187) -> ("Error Out"=w192:errorcluster, "time string"=w190:string, "date string"=w191:string)  [unwired: 8 in]
          n29 = call "AlliGator Format Script Output.vi"("Array of Simulation Outputs"=w181) -> ("Simulation Output String"=w180:string)  [unwired: 9 in, 1 out]
          n30 = Format Into String(format string="Script ended on %s at %s.\nFormatted script output:\n----------------------------\n%s", error in=w192, w191, w190, w180) -> (resulting string=w189:string, error out=w185:errorcluster)  [unwired: 1 in]
          n31 = global write "AlliGator FMB Global.vi" "Abort"(w179) -> ()
        }
        frame "Export Results" {
          n32 = local read "Decay Fit Options"() -> (w211:T9)
          n33 = local read "MLE Baseline Offset Type"() -> (w208:T6)
          n34 = local read "MLE Baseline Offset"() -> (w207:dbl)
          n35 = local read "Fit Parameter Constraints"() -> (w210:T7[])
          n36 = local read "Use Experimental IRF"() -> (w209:bool)
          n37 = Bundle("Decay Fit Options"=w211, "Fit Parameter Constraints"=w210, "Use Experimental IRF"=w209, "MLE Baseline Offset Type"=w208, "MLE Baseline Offset"=w207) -> (w205:T29)  [unwired: 1 in]
          n38 = call "AlliGator Save Simulation Outputs to ASCII.vi"("Fit Settings"=w205, "Simulation Parameters Array"=w206, "Fit Results"=w220) -> ("Error Out"=w221:errorcluster, "Message"=w212:string)  [unwired: 7 in]
        }
        frame "Graph Event" {
          n39 = Variant To Data(type=T25 {"Item Tag"="", "XY Graph Refnum"=refnum, "Coords"={"Horizontal"=0, "Vertical"=0}, "Item Path"=""} ("XY Graph Event"), Variant=w237) -> (data=w235:T25)  [unwired: 1 in, 1 out]
          n40 = Unbundle By Name(w235) -> ("XY Graph Refnum"=w233:refnum<vi>, "Item Tag"=w234:string)
          n41 = case shown="\"\", Default" w234 {
            tunnel: [w255 _ w270] -> w246
            tunnel: [w256 w258 w269] -> w245
            tunnel: w242 -> [w252 w259 w268]
            tunnel: [w251 w259 w268] -> w241
            tunnel: w240 -> [w253 w260 w267]
            tunnel: [w254 w260 w267] -> w238
            tunnel: w235 -> [_ _ w266]
            tunnel: w233 -> [w250 w257 _]
            tunnel: [_ _ w265] -> w232
            frame "Load Experimental IRF" {
              n42 = call "AlliGator Load Experimental IRF.vi"("Experimental IRF Loaded?"=w253, "Plot Data in"=w252, "XYGraph in"=w250) -> ("error out"=w256:errorcluster, "Experimental IRF Loaded?"=w254:bool, "Plot Data out"=w251:T30, "Message"=w255:string)  [unwired: 5 in]
            }
            frame "Show Experimental IRF" {
              n43 = case shown="True" w260 {
                tunnel: w259 -> [_ w264]
                tunnel: w257 -> [_ w263]
                tunnel: [_ w261] -> w258
                frame False {
                }
                frame True {
                  n44 = call-poly "XY Graph Add Plot(s) with Name(s).vi"("XYGraph Ref in"=w263, "Plot"=w264, "Plot Name (\"Plot\")"="Experimental IRF" ("Plot Name (\"Plot\")")) -> ("error out"=w261:errorcluster)  [unwired: 9 in, 3 out]
                }
              }
            }
            frame "", Default {
              n45 = call "XY Graph Special Event Handler Core.vi"("XY Graph Event"=w266) -> ("error out"=w269:errorcluster, "Message"=w270:string, "Message Type"=w265:T27)  [unwired: 5 in, 3 out]
            }
          }
        }
        frame "Idle", Default {
        }
        frame "Initialization" {
          n46 = vi-ref "Notebook.vi"() -> (w289:refnum<vi>)
          n47 = property class="VI"(reference=w289) -> (reference out=w292:refnum<vi>, error out=w291:errorcluster, "Path"=w290:path)  [unwired: 1 in]
          n48 = Close Reference(reference=w292, error in (no error)=w291) -> (error out=w293:errorcluster)
          n49 = call "Run Vi.vi"("VI Path"=w290, "error in (no error)"=w293, "Start Hidden? (F)"=TRUE) -> ()  [unwired: 5 in, 2 out]
        }
        frame "Quit" {
          w319 = dbl[] [] ("tau 1")
          n50 = call "Destroy Embedded Progress Bar.vi"("Progress Bar Queue in"=w318) -> ()  [unwired: 10 in, 1 out]
        }
        frame "Run Script" {
          w326 = TRUE ("Visible")
          n51 = local read "Simulation Parameters Multiplication Factor (s)"() -> (w336:T16)
          n52 = local read "Simulation Parameters Increment(s)"() -> (w337:T17)
          n53 = local read "Decay Simulation Parameters"() -> (w340:T4)
          n54 = local read "Fit Simulation Parameters"() -> (w339:T3)
          n55 = local read "Parameter Set Choice"() -> (w342:T18)
          n56 = local read "Simulation Parameters"() -> (w341:T17[])
          n57 = local read "Use Experimental IRF"() -> (w324:bool)
          n58 = local read "# Steps"() -> (w338:i32)
          n59 = case shown="\"Parameter x Factor\"" w342 {
            tunnel: w341 -> [w349 _ _]
            tunnel: [w349 w351 w358] -> w333
            tunnel: w340 -> [_ w354 w360]
            tunnel: w339 -> [_ w353 w359]
            tunnel: w338 -> [_ w355 w361]
            tunnel: w337 -> [_ w352 _]
            tunnel: w336 -> [_ _ w357]
            tunnel: w324 -> [_ w350 w356]
            frame "User-provided Array", Default {
            }
            frame "Parameter Increment" {
              n60 = call "AlliGator Get Simulation Parameters (by Increment).vi"("Use Experimental IRF"=w350, "Simulation Parameters Increment"=w352, "Fit Simulation Parameters"=w353, "Decay Simulation Parameters"=w354, "# Steps"=w355) -> ("Simulation Parameters Array"=w351:T17[])  [unwired: 6 in]
            }
            frame "Parameter x Factor" {
              n61 = call "AlliGator Get Simulation Parameters (by x Factor).vi"("Use Experimental IRF"=w356, "Simulation Parameters x Factor"=w357, "Fit Simulation Parameters"=w359, "Decay Simulation Parameters"=w360, "# Steps"=w361) -> ("Simulation Parameters Array"=w358:T17[])  [unwired: 6 in]
            }
          }
          n62 = call "Show Animated Busy Icon with Message and Abort Button.vi"("Message"=w327, "Target VI reference"=w328) -> ("Error Out"=w329:errorcluster)  [unwired: 17 in]
          n63 = Array Size(array=w333) -> (size(s)=w332:i32)
          n64 = call "AlliGator FMB Run Script.vi"("Error In"=w329, "# Steps"=w332, "FMB Q Elements in"=w335) -> ("Error Out"=w330:errorcluster, "Array of Simulation Outputs"=w321:T28[], "FMB Q Elements out"=w334:T22[], "Message"=w331:string)  [unwired: 5 in]
        }
        frame "Run Simulation" {
          w404 = TRUE  # New Simulation
          n65 = local read "Decay Simulation Parameters"() -> (w371:T4)
          n66 = local read "Fit Parameter Constraints"() -> (w388:T7[])
          n67 = local read "MLE Baseline Offset Type"() -> (w386:T6)
          n68 = local read "Plot Decays, Fits & Residuals"() -> (w391:bool)
          n69 = local read "Fit Simulation Parameters"() -> (w372:T3)
          n70 = local read "Use Experimental IRF"() -> (w370:bool)
          n71 = local read "MLE Baseline Offset"() -> (w387:dbl)
          n72 = local read "Decay Fit Options"() -> (w389:T9)
          n73 = Unbundle By Name(w389) -> ("Period"=w398:dbl[unit])
          n74 = Select(t=w403, s=w370, f=w402) -> (s? t:f=w393:T30)
          n75 = call "Show Animated Busy Icon with Message and Abort Button.vi"("Already active? (F)"=w380, "Target VI reference"=w406, "Error In"=errorcluster {"status"=FALSE, "code"=0, "source"=""}) -> ("Error Out"=w399:errorcluster)  [unwired: 16 in]
          n76 = Bundle By Name(cluster=T20 {"SYNC Period"=0.0, "Fit Options"={"Show Fit Residuals"=FALSE, "Fit Model"=enum."1-Exponential", "Residual Type"=enum."Standard", "Max Decay Percentile"=0.0, "Min Decay Percentile"=0.0, "Show Full Decay"=FALSE, "Weights"=enum."Unweighted", "Fitting Method"=enum."Least Square", "Compute Parameter Uncertainties"=FALSE, "Periodic Boundaries"=FALSE, "Model Calculation"=enum."Simulation", "Period"=0.0, "Termination Criteria"={"Max Iterations"=0, "Max Function Calls"=0, "Max Time"=0.0, "Function Tolerance"=0.0, "Parameter Tolerance"=0.0, "Gradient Tolerance"=0.0, "Min Lambda"=0.0, "Max Lambda"=0.0, "Initial Tick Count"=0}, "Offset Resolution"=0.0, "Use Local IRF"=FALSE, "Fitting Algorithm"=enum."Levenberg-Marquardt", "Show Confidence Interval "=TRUE, "Confidence Level"=95.0}, "Fit Parameter Constraints"=[], "MLE Baseline Offset"=0.0, "MLE Baseline Offset Type"=enum."Absolute"} ("Decay Fit Options & Parameters"), "Fit Options"=w389, "SYNC Period"=w398, "Fit Parameter Constraints"=w388, "MLE Baseline Offset"=w387, "MLE Baseline Offset Type"=w386) -> (w367:T20)
          n77 = Bundle By Name(cluster=T17 {"Decay Simulation Parameters"={"tau 1"=1e-09, "tau 2"=0.0, "a1"=1.0, "Baseline"=0.0}, "Fit Simulation Parameters"={"# Counts"=100, "# Simulations (N)"=100, "Decay Bin Size"=1.0000000000000002e-10, "# Bins"=200}, "Use Experimental IRF"=FALSE} ("Simulation Parameters"), "Use Experimental IRF"=w370, "Fit Simulation Parameters"=w372, "Decay Simulation Parameters"=w371) -> (w368:T17)
          n78 = call "AlliGator Fit Linear Combinations of Exponentials.vi"("Simulation Parameters"=w368, "Decay Fit Options & Parameters"=w367, "Reference Decay"=w393, "Error In"=w399, "Show Decays, Fits & Residuals"=w391) -> ("Output Plots"=w392:cluster{"t Array":dbl[], "I Array":dbl[]}[], "Output Plot Names"=w395:string[], "Plot Colors"=w385:u32[], "Fit Results"=w377:T31[], "tau 1"=w411:dbl[], "tau 2"=w410:dbl[], "a 1"=w409:dbl[], "Message"=w408:string, "Error Out"=w396:errorcluster)  [unwired: 2 in]
          n79 = call "AlliGator Decay Sum.vi"("Output Plots"=w392) -> ("# Photons"=w390:dbl[])
          n80 = local write "# Photons"(w390) -> ()
          n81 = call "XY Graph Add Multiplots with Names v2.vi"("XYGraph in"=w405, "Keep Existing Plots (T)"=FALSE, "Array of Plots"=w392, "Array of Plot Names (\"Plot\")"=w395, "error in (no error)"=w396, "Plot Colors (Default)"=w385) -> ("error out"=w379:errorcluster)  [unwired: 5 in, 4 out]
          n82 = Bundle By Name(cluster=T19 {"Simulation Parameters"={"Decay Simulation Parameters"={"tau 1"=0.0, "tau 2"=0.0, "a1"=0.0, "Baseline"=0.0}, "Fit Simulation Parameters"={"# Counts"=0, "# Simulations (N)"=0, "Decay Bin Size"=0.0, "# Bins"=0}, "Use Experimental IRF"=FALSE}, "Decay Fit Options & Parameters"={"SYNC Period"=0.0, "Fit Options"={"Show Fit Residuals"=FALSE, "Fit Model"=enum."1-Exponential", "Residual Type"=enum."Standard", "Max Decay Percentile"=0.0, "Min Decay Percentile"=0.0, "Show Full Decay"=FALSE, "Weights"=enum."Unweighted", "Fitting Method"=enum."Least Square", "Compute Parameter Uncertainties"=FALSE, "Periodic Boundaries"=FALSE, "Model Calculation"=enum."Simulation", "Period"=0.0, "Termination Criteria"={"Max Iterations"=0, "Max Function Calls"=0, "Max Time"=0.0, "Function Tolerance"=0.0, "Parameter Tolerance"=0.0, "Gradient Tolerance"=0.0, "Min Lambda"=0.0, "Max Lambda"=0.0, "Initial Tick Count"=0}, "Offset Resolution"=0.0, "Use Local IRF"=FALSE, "Fitting Algorithm"=enum."Levenberg-Marquardt", "Show Confidence Interval "=FALSE, "Confidence Level"=0.0}, "Fit Parameter Constraints"=[], "MLE Baseline Offset"=0.0, "MLE Baseline Offset Type"=enum."Absolute"}} ("output cluster"), "Simulation Parameters"=w368, "Decay Fit Options & Parameters"=w367) -> (w365:T19)
          n83 = Bundle("Fit Results"=w377) -> (w376:cluster{"Fit Results":T31[]})  [unwired: 1 in]
          n84 = case shown="True" w378 {
            tunnel: w376 -> [w413 w415]
            tunnel: [w412 w414] -> w375
            tunnel: w374 -> [_ w416]
            frame False {
              n85 = Build Array(w413) -> (w412:cluster{"Fit Results":T31[]}[])
            }
            frame True {
              n86 = Build Array (concatenate)(w416, w415) -> (w414:cluster{"Fit Results":T31[]}[])
            }
          }
          n87 = Build Array (concatenate)(T22 {"FMB Q Event"=enum."Update Histograms", "Data"=variant} ("element"), w384) -> (w383:T22[])
          n88 = call "Hide Animated Busy Icon with Message and Abort Button.vi"("Already active? (F)"=w380, "Message"=w408, "Target VI reference"=w406, "Error In"=w379) -> ("Error Out"=w407:errorcluster)  [unwired: 15 in]
        }
        frame "Show Selected Decay" {
          n89 = call-poly "Variant to Data.vi"("Variant"=w423) -> ("Value"=w425:i32)  [unwired: 8 in]
          n90 = Decrement(x=w425) -> (x-1=w431:i32)
          n91 = Multiply(x=w431, y=3) -> (x*y=w428:i32)
          n92 = Increment(x=w428) -> (x+1=w427:i32)
          n93 = Increment(x=w427) -> (x+1=w426:i32)
          n94 = Build Array(w428, w427, w426) -> (w429:i32[])
          n95 = call "XY Graph Set Selected Plots.vi"("Selected Plots"=w429, "XY Graph Refnum"=w436) -> ()  [unwired: 6 in, 4 out]
        }
        frame "Single Simulation Prelude" {
          n96 = local read "Decay Simulation Parameters"() -> (w446:T4)
          n97 = local read "Fit Simulation Parameters"() -> (w445:T3)
          n98 = Bundle By Name(cluster=T17 {"Decay Simulation Parameters"={"tau 1"=0.0, "tau 2"=0.0, "a1"=0.0, "Baseline"=0.0}, "Fit Simulation Parameters"={"# Counts"=0, "# Simulations (N)"=0, "Decay Bin Size"=0.0, "# Bins"=0}, "Use Experimental IRF"=FALSE} ("Simulation Parameters Increment"), "Decay Simulation Parameters"=w446, "Fit Simulation Parameters"=w445) -> (w448:T17)
          n99 = Build Array(w448) -> (w447:T17[])
        }
        frame "Update # Processors Used" {
          n100 = call-poly "Variant to Data.vi"("Variant"=w468) -> ("Value"=w467:i32)  [unwired: 8 in]
          n101 = call "Logical Processors Used.vi"("Set/Get (F)"=TRUE, "# Logical Processor Used"=w467) -> ()  [unwired: 4 in, 1 out]
          n102 = call "IMAQ Multi-Core Options"("Get/Set Number of Cores (Get)"=enum32{"Get", "Set", "Set Max Available"}."Set", "Specified Number of Cores"=w467) -> ()  [unwired: 8 in, 2 out]
        }
        frame "Update Histograms" {
          n103 = local read "Histogram Options"() -> (w479:T2)
          n104 = call "Is Value Changed.vim"("value"=w505) -> ("changed or first call?"=w491:bool)
          n105 = call "Is Value Changed.vim"("value"=w507) -> ("changed or first call?"=w493:bool)
          n106 = call "Is Value Changed.vim"("value"=w506) -> ("changed or first call?"=w492:bool)
          n107 = Compound Arithmetic op=OR(w493, w492, w491) -> (invert w490:bool)
          n108 = Empty Array?(array=w507) -> (empty?=w494:bool)
          n109 = case shown="False" w494 {
            tunnel: w506 -> [w525 _]
            tunnel: w505 -> [w524 _]
            tunnel: w507 -> [w523 _]
            tunnel: [w522 _] -> w489
            tunnel: [w518 _] -> w503
            tunnel: w502 -> [w521 _]
            tunnel: w500 -> [w516 _]
            tunnel: w483 -> [w514 _]
            tunnel: [w509 w541] -> w482
            tunnel: w481 -> [_ w541]
            tunnel: w479 -> [w508 _]
            frame False {
              n110 = call "AlliGator Compute Lifetime Simulation Histograms.vi"("tau 1"=w523, "tau 2"=w525, "a1"=w524, "Histogram Options"=w508) -> ("Histograms"=w520:cluster{"Axis":dbl[], "Histogram":dbl[]}[], "Array Statistic (tau 1)"=w513:T5, "Array Statistics (tau 2)"=w511:T5, "Array Statistics (a1)"=w512:T5, "Array of Scales"=w515:cluster{"X Scale":u32, "Y Scale":u32}[], "Plot Names"=w517:string[], "Message"=w522:string, "Error Out"=w519:errorcluster)  [unwired: 4 in]
              n111 = Bundle By Name(cluster=T28 {"Simulation & Fit Options & Parameters"={"Simulation Parameters"={"Decay Simulation Parameters"={"tau 1"=0.0, "tau 2"=0.0, "a1"=0.0, "Baseline"=0.0}, "Fit Simulation Parameters"={"# Counts"=0, "# Simulations (N)"=0, "Decay Bin Size"=0.0, "# Bins"=0}, "Use Experimental IRF"=FALSE}, "Decay Fit Options & Parameters"={"SYNC Period"=0.0, "Fit Options"={"Show Fit Residuals"=FALSE, "Fit Model"=enum."1-Exponential", "Residual Type"=enum."Standard", "Max Decay Percentile"=0.0, "Min Decay Percentile"=0.0, "Show Full Decay"=FALSE, "Weights"=enum."Unweighted", "Fitting Method"=enum."Least Square", "Compute Parameter Uncertainties"=FALSE, "Periodic Boundaries"=FALSE, "Model Calculation"=enum."Simulation", "Period"=0.0, "Termination Criteria"={"Max Iterations"=0, "Max Function Calls"=0, "Max Time"=0.0, "Function Tolerance"=0.0, "Parameter Tolerance"=0.0, "Gradient Tolerance"=0.0, "Min Lambda"=0.0, "Max Lambda"=0.0, "Initial Tick Count"=0}, "Offset Resolution"=0.0, "Use Local IRF"=FALSE, "Fitting Algorithm"=enum."Levenberg-Marquardt", "Show Confidence Interval "=FALSE, "Confidence Level"=0.0}, "Fit Parameter Constraints"=[], "MLE Baseline Offset"=0.0, "MLE Baseline Offset Type"=enum."Absolute"}}, "Array Statistic (tau 1)"={"Mean"=0.0, "Standard Deviation"=0.0, "Max"=0.0, "Min"=0.0}, "Array Statistics (a1)"={"Mean"=0.0, "Standard Deviation"=0.0, "Max"=0.0, "Min"=0.0}, "Array Statistics (tau 2)"={"Mean"=0.0, "Standard Deviation"=0.0, "Max"=0.0, "Min"=0.0}} ("Simulation Output"), "Simulation & Fit Options & Parameters"=w514, "Array Statistic (tau 1)"=w513, "Array Statistics (a1)"=w512, "Array Statistics (tau 2)"=w511) -> (w509:T28)
              n112 = local write "tau 1"(w513) -> ()
              n113 = local write "tau 2"(w511) -> ()
              n114 = local write "a1"(w512) -> ()
              n115 = case shown="True" w516 {
                tunnel: w521 -> [w532 w540]
                tunnel: w520 -> [w531 w539]
                tunnel: w519 -> [w529 w538]
                tunnel: [w528 w537] -> w518
                tunnel: w517 -> [w530 w536]
                tunnel: w515 -> [w526 w535]
                frame False {
                  n116 = call "XY Graph Replace Multiplots with Names.vi"("XYGraph in"=w532, "Array of Scales (Default)"=w526, "Array of Plots"=w531, "Array of Plot Names (\"Plot\")"=w530, "error in (no error)"=w529, "Make Visible (T)"=TRUE) -> ("error out"=w528:errorcluster)  [unwired: 5 in, 4 out]
                }
                frame True {
                  n117 = call "XY Graph Add Multiplots with Names v2.vi"("XYGraph in"=w540, "Array of Scales (Default)"=w535, "Array of Plots"=w539, "Array of Plot Names (\"Plot\")"=w536, "error in (no error)"=w538, "Make Visible (T)"=TRUE, "Plot Colors (Default)"=u32[] [0, 16711680, 65280]) -> ("error out"=w537:errorcluster)  [unwired: 4 in, 4 out]
                }
              }
            }
            frame True {
            }
          }
          n118 = Select(t="", s=w490, f=w489) -> (s? t:f=w504:string)
          n119 = call "AlliGator Too Many Histogram Bins Message.vi"("error in (no error)"=w503) -> ()
        }
        frame "Update Script Simulation Parameters" {
          n120 = Index Array(array=w546, index=w542) -> (element=w550:T17)
          n121 = Unbundle By Name(w550) -> ("Decay Simulation Parameters"=w548:T4, "Fit Simulation Parameters"=w549:T3)
          n122 = local write "Decay Simulation Parameters"(w548) -> ()
          n123 = local write "Fit Simulation Parameters"(w549) -> ()
        }
        frame "Update Script Simulation Output" {
          n124 = Increment(x=w561) -> (x+1=w560:i32)
          n125 = Replace Array Subset(array=w564, new element=w562, index=w561) -> (w563:T28[])
        }
      }
      n126 = call "Get Current Message Text Format.vi"("Text Format"=w112) -> ("Message Formatting"=w113:T32)  [unwired: 8 in, 1 out]
      n127 = local write "Experimental IRF Loaded"(w109) -> ()
      n128 = Empty Array?(array=w104) -> (empty?=w106:bool)
      n129 = call "Send Message to Notebook.vi"("Text Formatting"=w113, "Error In"=w125, "Text"=w129, "Notebook Queue"=w130) -> ("Error Out"=w127:errorcluster, "Notebook Queue"=w128:refnum<queue>)  [unwired: 4 in]
      n130 = call "Send Error to Notebook.vi"("error in (no error)"=w127, "Notebook Q"=w128) -> ("Error Out"=w126:errorcluster)  [unwired: 9 in]
    }
    n131 = call "Tiny Clear Error.vi"("Error In"=w80) -> ("no Error Out"=w79:errorcluster)  [unwired: 8 in]
  }
  n132 = call "XY Graph TipStrip Event Registration.vi"("XY Graph Refnum"=w24) -> ("Event Registration Refnum"=w22:refnum<event-registration>)  [unwired: 8 in, 2 out]
  n133 = call "XY Graph TipStrip Event Registration.vi"("XY Graph Refnum"=w23) -> ("Event Registration Refnum"=w21:refnum<event-registration>)  [unwired: 8 in, 2 out]
  n134 = Enqueue Element(queue=w15, element=w4, error in (no error)=w3) -> (queue out=w5:refnum<queue>)  [unwired: 1 in, 2 out]
  n135 = Bundle(cluster=T23 {"Decay Graph"=refnum, "Histograms"=refnum}, "Decay Graph"=w22, "Histograms"=w21) -> (w14:T23)
  n136 = CPU Information() -> (4:w30:i32)  [unwired: 3 out]
  "# Logical Processors" <- w30
  n137 = call "Logical Processors Used.vi"("Set/Get (F)"=TRUE, "# Logical Processor Used"=w30) -> ()  [unwired: 4 in, 1 out]
  n138 = while {
    tunnel: w5 -> [w581]
    tunnel: w14 -> [w580]
    tunnel: [w579] -> w13
    stop <- w582 stop-if-true
    # "Event Loop"
    n139 = event shown="[14] <Histograms.XY Graph Refnum>: Mouse Leave" {
      selector: w580 -> [_ _ _ _ _ _ _ _ _ _ _ _ w639 w647 w652 w654 _ _ _]
      dyn-events: [_ _ _ _ _ _ _ _ _ _ _ _ w638 w646 w651 w653 _ _ _] -> w579
      timeout: _ -> [_ _ _ _ _ _ _ _ _ _ _ _ _ _ _ _ _ _ _]
      tunnel: [w586 w588 _ _ _ _ _ _ _ _ _ _ _ _ _ _ _ _ _] -> w582
      tunnel: [T22[] [{"FMB Q Event"=enum."Quit", "Data"=variant}] ("element") w589 _ _ T22[] [{"FMB Q Event"=enum."Abort", "Data"=variant}] ("element") T22[] [{"FMB Q Event"=enum."Single Simulation Prelude", "Data"=variant}, {"FMB Q Event"=enum."Run Simulation", "Data"=variant}] ("element") T22[] [{"FMB Q Event"=enum."Run Script", "Data"=variant}] ("element") T22[] [{"FMB Q Event"=enum."Export Results", "Data"=variant}] ("element") w620 T22[] [{"FMB Q Event"=enum."Update Histograms", "Data"=variant}] ("element") w630 w634 _ _ _ _ _ _ w664] -> w578
      event Panel Close? {
        w586 = TRUE ("Discard?")
        n140 = event-data() -> ()  [unwired: 1 in, 1 out]
        n141 = event-data("Discard?"=w586) -> ()  [unwired: 1 in, 1 out]
      }
      event Menu Selection (User) {
        n142 = event-data() -> ("MenuRef"=w587:refnum<k9>, "ItemTag"=w590:string)  [unwired: 1 in]
        n143 = case shown="\"Abort\"" w590 {
          selector: w590 -> [_ _ _ _ _ _ w598 _]
          tunnel: [_ T22[] [{"FMB Q Event"=enum."Quit", "Data"=variant}] ("element") T22[] [{"FMB Q Event"=enum."Export Results", "Data"=variant}] ("element") T22[] [{"FMB Q Event"=enum."Run Script", "Data"=variant}] ("element") T22[] [{"FMB Q Event"=enum."Abort", "Data"=variant}] ("element") T22[] [{"FMB Q Event"=enum."Single Simulation Prelude", "Data"=variant}, {"FMB Q Event"=enum."Run Simulation", "Data"=variant}] ("element") _ _] -> w589
          tunnel: [_ TRUE ("Discard?") _ _ _ _ _ _] -> w588
          tunnel: w587 -> [_ _ _ _ _ _ w599 _]
          frame "", Default {
          }
          frame "Quit" {
          }
          frame "Export Results" {
          }
          frame "Run Script" {
          }
          frame "Abort" {
            n144 = global write "AlliGator FMB Global.vi" "Abort"(TRUE ("Abort")) -> ()
          }
          frame "Run Simulation" {
          }
          frame "Plot Decays, Fits & Residuals" {
            n145 = local read "Plot Decays, Fits & Residuals"() -> (w601:bool)
            n146 = Not(x=w601) -> (.not. x?=w600:bool)
            n147 = local write "Plot Decays, Fits & Residuals"(w600) -> ()
            n148 = Set Menu Item Info(6:w600, 7:w598, 10:w598, 11:w599) -> ()  [unwired: 3 in, 2 out]
          }
          frame "Show Notebook" {
            n149 = vi-ref "Notebook.vi"() -> (w607:refnum<vi>)
            n150 = property class="VI"(reference=w607) -> (reference out=w604:refnum<vi>, error out=w605:errorcluster, "Path"=w606:path)  [unwired: 1 in]
            n151 = Close Reference(reference=w604, error in (no error)=w605) -> (error out=w603:errorcluster)
            n152 = call "Run Vi.vi"("VI Path"=w606, "error in (no error)"=w603, "Start Hidden? (F)"=TRUE) -> ()  [unwired: 5 in, 2 out]
          }
        }
      }
      event "Parameter Set Choice": Value Change {
        n153 = event-data() -> ("NewVal"=w609:T18)  [unwired: 1 in]
        n154 = case shown="\"Parameter Increment\", Default" w609 {
          tunnel: [FALSE ("Visible") TRUE ("Visible")] -> w608
          frame "User-provided Array" {
          }
          frame "Parameter Increment", Default {
          }
        }
        n155 = property on="# Steps" class="DigNum (strict)"("Visible"=w608) -> ()  [unwired: 2 in, 2 out]
      }
      event Menu Activation? {
        w613 = "Plot Decays, Fits & Residuals" ("item tag")
        n156 = event-data() -> ("MenuRef"=w614:refnum<k9>)  [unwired: 1 in]
        n157 = local read "Plot Decays, Fits & Residuals"() -> (w612:bool)
        n158 = Set Menu Item Info(6:w612, 7:w613, 10:w613, 11:w614) -> ()  [unwired: 3 in, 2 out]
        n159 = event-data() -> ()  [unwired: 2 in, 1 out]
      }
      event "Abort": Value Change {
        n160 = event-data() -> ()  [unwired: 1 in, 1 out]
        n161 = global write "AlliGator FMB Global.vi" "Abort"("Abort") -> ()
      }
      event "Run Simulation": Value Change {
        n162 = event-data() -> ()  [unwired: 1 in, 1 out]
      }
      event "Run Script": Value Change {
        n163 = event-data() -> ()  [unwired: 1 in, 1 out]
      }
      event "Export Results": Value Change {
        n164 = event-data() -> ()  [unwired: 1 in, 1 out]
      }
      event "Histograms", "Decay Graph": Shortcut Menu Selection (User) {
        n165 = event-data() -> ("ItemTag"=w626:string, "CtlRef"=w625:refnum<vi>, "Coords"=w624:T26, "ItemPath"=w623:string)  [unwired: 1 in]
        n166 = Bundle By Name(cluster=T25 {"Item Tag"="", "XY Graph Refnum"=refnum, "Coords"={"Horizontal"=0, "Vertical"=0}, "Item Path"=""} ("XY Graph Event"), "Item Tag"=w626, "XY Graph Refnum"=w625, "Coords"=w624, "Item Path"=w623) -> (w621:T25)
        n167 = Bundle By Name(cluster=T22 {"FMB Q Event"=enum."Graph Event", "Data"=variant} ("element"), "Data"=w621) -> (w622:T22)
        n168 = Build Array(w622) -> (w620:T22[])
      }
      event Value Change {
        n169 = event-data() -> ()  [unwired: 1 in, 1 out]
      }
      event "Select Decay, Fit & Residuals Index": Value Change {
        n170 = event-data() -> ("NewVal"=w631:i32)  [unwired: 1 in]
        n171 = Bundle By Name(cluster=T22 {"FMB Q Event"=enum."Show Selected Decay", "Data"=variant} ("element"), "Data"=w631) -> (w632:T22)
        n172 = Build Array(w632) -> (w630:T22[])
      }
      event Value Change {
        n173 = event-data() -> ("NewVal"=w635:dbl)  [unwired: 1 in]
        n174 = Bundle By Name(cluster=T22 {"FMB Q Event"=enum."Check Baseline", "Data"=variant} ("element"), "Data"=w635) -> (w636:T22)
        n175 = Build Array(w636) -> (w634:T22[])
      }
      event Mouse Enter {
        n176 = event-data() -> ("CtlRef"=w640:refnum<vi>)  [unwired: 1 in]
        n177 = Unbundle By Name(w639) -> ("Decay Graph"=w641:refnum<event-registration>)
        n178 = call "XY Graph Tipstrip Mouse Enter.vi"("Event Registration Refnum"=w641, "XY Graph Refnum"=w640) -> ("Event Registration Refnum"=w642:refnum<event-registration>)  [unwired: 8 in, 1 out]
        n179 = Bundle By Name(cluster=w639, "Decay Graph"=w642) -> (w638:T23)
      }
      event Mouse Leave {
        n180 = event-data() -> ("CtlRef"=w645:refnum<vi>)  [unwired: 1 in]
        n181 = Unbundle By Name(w647) -> ("Decay Graph"=w644:refnum<event-registration>)
        n182 = call "XY Graph Tipstrip Mouse Leave.vi"("Event Registration Refnum"=w644, "XY Graph Refnum"=w645) -> ("Event Registration Refnum"=w643:refnum<event-registration>)  [unwired: 8 in, 1 out]
        n183 = Bundle By Name(cluster=w647, "Decay Graph"=w643) -> (w646:T23)
      }
      event Mouse Leave {
        n184 = event-data() -> ("CtlRef"=w650:refnum<vi>)  [unwired: 1 in]
        n185 = Unbundle By Name(w652) -> ("Histograms"=w649:refnum<event-registration>)
        n186 = call "XY Graph Tipstrip Mouse Leave.vi"("Event Registration Refnum"=w649, "XY Graph Refnum"=w650) -> ("Event Registration Refnum"=w648:refnum<event-registration>)  [unwired: 8 in, 1 out]
        n187 = Bundle By Name(cluster=w652, "Histograms"=w648) -> (w651:T23)
      }
      event Mouse Enter {
        n188 = event-data() -> ("CtlRef"=w655:refnum<vi>)  [unwired: 1 in]
        n189 = Unbundle By Name(w654) -> ("Histograms"=w656:refnum<event-registration>)
        n190 = call "XY Graph Tipstrip Mouse Enter.vi"("Event Registration Refnum"=w656, "XY Graph Refnum"=w655) -> ("Event Registration Refnum"=w657:refnum<event-registration>)  [unwired: 8 in, 1 out]
        n191 = Bundle By Name(cluster=w654, "Histograms"=w657) -> (w653:T23)
      }
      event Mouse Move {
        n192 = event-data() -> ("CtlRef"=w658:refnum<vi>, "Coords"=w659:T26)  [unwired: 1 in]
        n193 = control-ref of="Decay Graph ToolTip"() -> (w660:refnum<vi>)
        n194 = call "XY Graph Set Plot TipStrip.vi"("TipStrip Refnum"=w660, "Coords"=w659, "XY Graph Refnum"=w658) -> ()  [unwired: 6 in, 3 out]
      }
      event Mouse Move {
        n195 = event-data() -> ("CtlRef"=w661:refnum<vi>, "Coords"=w662:T26)  [unwired: 1 in]
        n196 = control-ref of="Histograms ToolTip"() -> (w663:refnum<vi>)
        n197 = call "XY Graph Set Plot TipStrip.vi"("TipStrip Refnum"=w663, "Coords"=w662, "XY Graph Refnum"=w661) -> ()  [unwired: 6 in, 3 out]
      }
      event "# Logical Processors Used": Value Change {
        n198 = event-data() -> ("NewVal"=w665:i32)  [unwired: 1 in]
        n199 = Bundle By Name(cluster=T22 {"FMB Q Event"=enum."Update # Processors Used", "Data"=variant} ("element"), "Data"=w665) -> (w666:T22)
        n200 = Build Array(w666) -> (w664:T22[])
      }
    }
    n201 = Array Size(array=w578) -> (size(s)=w577:i32)
    n202 = case shown="0" w577 {
      tunnel: w581 -> [_ w584]
      tunnel: w578 -> [_ w583]
      frame 0 {
      }
      frame 1, Default {
        n203 = Enqueue Element(queue=w584, element=w583) -> ()  [unwired: 2 in, 3 out]
      }
    }
  }
  n204 = property on="# Logical Processors Used" class="DigNum (strict)"("Maximum"=w30, "Minimum"=w28, "OutOfRngActMax"=w28, "OutOfRngActMin"=w28) -> ()  [unwired: 2 in, 2 out]
  n205 = while {
    tunnel: w9 -> [w673]
    tunnel: w45 -> [w671]
    tunnel: [w668] -> w44
    stop <- w669 stop-if-true
    n206 = Dequeue Element(queue=w673) -> (element=w672:T36, error out=w670:errorcluster)  [unwired: 2 in, 2 out]
    n207 = call "Update Embedded Progress Bar Indicator.vi"("Error In"=w670, "Progress Bar Event"=w672, "Progress Bar Refnum"=w671) -> ("Error Out"=w668:errorcluster, "Quit?"=w669:bool)  [unwired: 7 in]
  }
  n208 = Release Queue(queue=w9, force destroy? (F)=TRUE, error in (no error)=w44) -> (error out=w40:errorcluster)  [unwired: 2 out]
  n209 = call "Tiny Clear Error.vi"("Error In"=w40) -> ("no Error Out"=w25:errorcluster)  [unwired: 8 in]
  n210 = case shown="\"Simulations\", Default" "Tab Control" {
    frame "Simulations", Default {
    }
    frame "Decay, Fit & Residuals Plots" {
    }
    frame "Settings" {
    }
    frame "Scripts" {
    }
  }
  n211 = Unregister For Events(event registration refnum=w13) -> (error out=w10:errorcluster)  [unwired: 1 in]
  n212 = Release Queue(queue=w12) -> (error out=w11:errorcluster)  [unwired: 2 in, 2 out]
  n213 = Merge Errors(w41, w11, w10, w25) -> (w39:errorcluster)
  n214 = invoke class="VI" method="FP.Close"(reference=w36, error in=w39) -> (reference out=w38:refnum<vi>, error out=w37:errorcluster)  [unwired: 1 in, 1 out]
  n215 = Close Reference(reference=w38, error in (no error)=w37) -> ()  [unwired: 1 out]
